vi "Toast Drive.vi"(2 "Joy Y In":dbl, 3 "Joy X In":dbl) -> (0 "Speed Control Out":dbl, 1 "Angle Control Out":dbl)   [LabVIEW 2011]
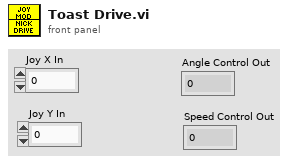
[diagram p1: front panel]
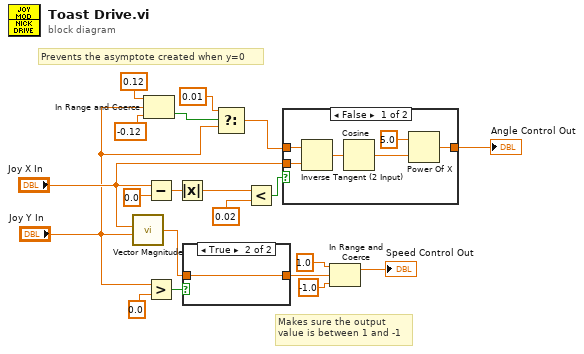
[diagram p0: block diagram]
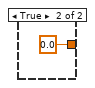
[diagram p2: hidden frame]
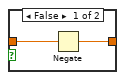
[diagram p3: hidden frame]
diagram:
  # "Prevents the asymptote created when y=0"
  # "Makes sure the output \nvalue is between 1 and -1"
  n1 = call "Vector Magnitude.vi"("X Component"="Joy X In", "Y Component"="Joy Y In") -> ("Magnitude"=w19:dbl)  [unwired: 6 in]
  n2 = In Range and Coerce(upper limit=0.12, x="Joy Y In", lower limit=-0.12) -> (In Range?=w4:bool)  [unwired: 1 out]
  n3 = Subtract(x="Joy X In", y=0.0) -> (x-y=w13:dbl)
  n4 = Greater?(x="Joy Y In", y=0.0) -> (0:w18:bool)
  n5 = Absolute Value(x=w13) -> (abs(x)=w10:dbl)
  n6 = case shown="True" w18 {
    tunnel: w19 -> [w22 w23]
    tunnel: [w21 w23] -> w17
    frame False {
      n7 = Negate(x=w22) -> (-x=w21:dbl)
    }
    frame True {
    }
  }
  n8 = Select(t=0.01, s=w4, f="Joy Y In") -> (s? t:f=w2:dbl)
  n9 = Less?(x=w10, y=0.02) -> (x < y?=w8:bool)
  n10 = case shown="False" w8 {
    tunnel: w2 -> [w27 _]
    tunnel: "Joy X In" -> [w26 _]
    tunnel: [w24 0.0] -> w7
    frame False {
      n11 = Inverse Tangent (2 Input)(1:w26, 2:w27) -> (0:w25:dbl)
      n12 = Cosine(x=w25) -> (cos(x)=w28:dbl)
      n13 = Power Of X(1:w28, 2:5.0 ("y")) -> (0:w24:dbl)
    }
    frame True {
    }
  }
  "Angle Control Out" <- w7
  n14 = In Range and Coerce(upper limit=1.0, x=w17, lower limit=-1.0) -> (coerced(x)=→"Speed Control Out":dbl)  [unwired: 1 out]
